vi "_FPGA_AuxCycCalculator.vi"(6 "AuxIniCyc":u64, 8 "Init":bool, 9 "Scale*2^26":u32, 11 "PriRFCyc_U64":u64) -> (1 "AuxCyc":u64)   [LabVIEW 2018]
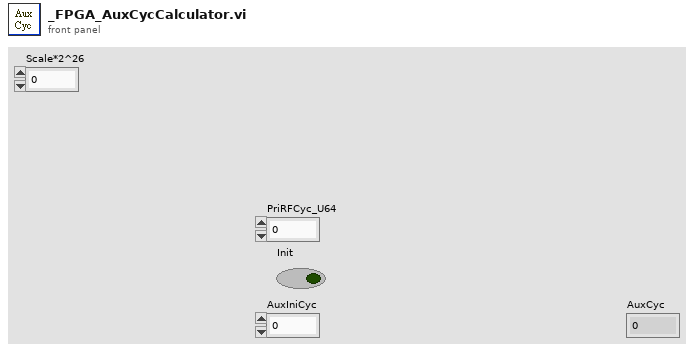
[diagram p1: front panel]
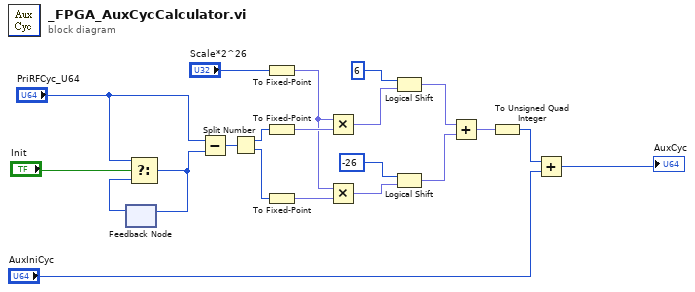
[diagram p0: block diagram]
diagram:
  n1 = feedback #1() -> (w20:u64)  [unwired: 1 in]
  n2 = Select(t="PriRFCyc_U64", s="Init", f=w20) -> (s? t:f=w19:u64)
  n3 = feedback-in #1(w19) -> ()
  n4 = Subtract(x="PriRFCyc_U64", y=w19) -> (x-y=w13:u64)
  n5 = Split Number(x=w13) -> (hi(x)=w12:u32, lo(x)=w11:u32)
  n6 = To Fixed-Point(number="Scale*2^26") -> (fixed-point=w9:fxp<+,32,32>)  [unwired: 1 in]
  n7 = To Fixed-Point(number=w12) -> (fixed-point=w10:fxp<+,32,32>)  [unwired: 1 in]
  n8 = To Fixed-Point(number=w11) -> (fixed-point=w8:fxp<+,32,32>)  [unwired: 1 in]
  n9 = Multiply(x=w9, y=w10) -> (x*y=w4:fxp<+,64,64>)
  n10 = Multiply(x=w9, y=w8) -> (x*y=w3:fxp<+,64,64>)
  n11 = Logical Shift(y=i16 6, x=w4) -> (x << y=w2:fxp<+,64,64>)
  n12 = Logical Shift(y=i16 -26, x=w3) -> (x << y=w5:fxp<+,64,64>)
  n13 = Add(x=w2, y=w5) -> (x+y=w6:fxp<+,64,64>)
  n14 = To Unsigned Quad Integer(1:w6) -> (0:w1:u64)
  n15 = Add(x=w1, y="AuxIniCyc") -> (x+y=→"AuxCyc":u64)
